vi "Auto Loop 5.vi"(2 "Auto State":u8, 3 "Call Context":T1) -> (1 "SubState 5":T2)   [LabVIEW 2013]
uses:
  typedefs/singleUseSubstate.ctl
  <vilib>/Rock Robotics/WPI/DriverStation/WPI_DriverStationDerivedRobotMode.ctl
  typedefs/subStates.ctl
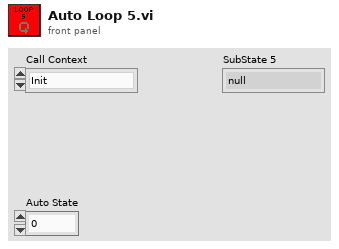
[diagram p1: front panel]
types:
  T1 = typedef "WPI_DriverStationDerivedRobotMode.ctl" = enum16{"Init", "Execute", "Stop"}
  T2 = typedef "singleUseSubstate.ctl" = enum16{"null", "wait", "shift high", "shift low"}
  T3 = typedef "subStates.ctl" = enum16{"null", "wait", "driver control", "auto", "manual override", "hold position", "rotate", "pickup", "pass", "load", "goto shoot", "shoot", "cancel", "end"}
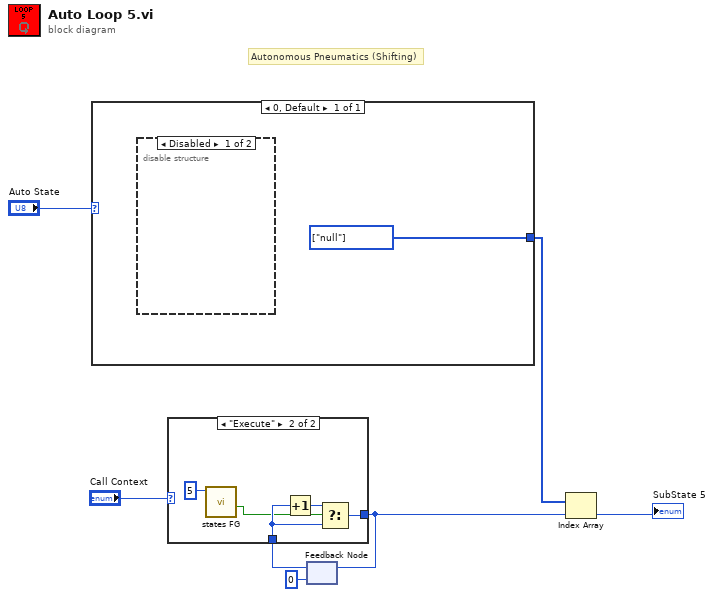
[diagram p0: block diagram]
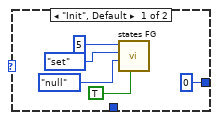
[diagram p2: hidden frame]
diagram:
  # "Autonomous Pneumatics (Shifting)"
  n1 = case shown="0, Default" "Auto State" {
    tunnel: [w8] -> w4
    frame 0, Default {
      w8 = T2[] [enum."null"] items=["null", "wait", "shift high", "shift low"]
      n2 = disable-structure shown="Disabled" {
        frame Disabled {
        }
        frame Enabled {
        }
      }
    }
  }
  n3 = feedback #1(0) -> (w7:i32)
  n4 = case shown="\"Execute\"" "Call Context" {
    tunnel: w7 -> [_ w17]
    tunnel: [0 w15] -> w5
    frame "Init", Default {
      n5 = call "states FG.vi"("exit in"=TRUE, "subState in"=subStates."null", "menu (get)"=enum16{"set", "get"}."set", "Loop ID"=5) -> ()  [unwired: 4 in, 4 out]
    }
    frame "Execute" {
      n6 = call "states FG.vi"("Loop ID"=5) -> ("exit out"=w14:bool)  [unwired: 7 in, 3 out]
      n7 = Increment(x=w17) -> (x+1=w16:i32)
      n8 = Select(t=w16, s=w14, f=w17) -> (s? t:f=w15:i32)
    }
  }
  n9 = feedback-in #1(w5) -> ()
  n10 = Index Array(array=w4, index=w5) -> (element=→"SubState 5":T2)
